vi "scale_matrix.vi"(1 "Scale Factors":cluster{dbl, dbl, dbl}) -> (0 "Scale Matrix":T1)   [LabVIEW 2019]
uses:
  <vilib>/Analysis/Matrix/Datatypes/RealMatrix.ctl
  <vilib>/Analysis/Matrix/Numeric/Conversions/Array To Matrix - RA2.vi
  <vilib>/Analysis/Matrix/NI_Matrix.lvlib
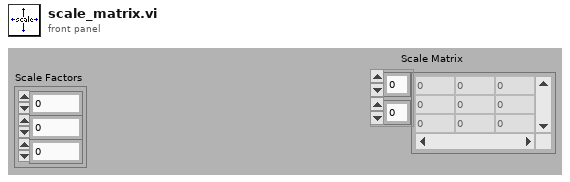
[diagram p1: front panel]
types:
  T1 = typedef "NI_Matrix.lvlib/RealMatrix.ctl" = dbl[][]
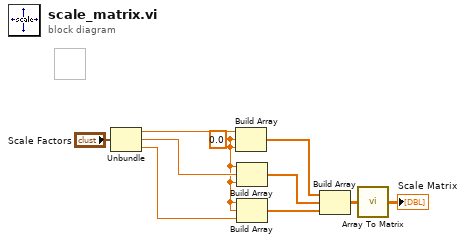
[diagram p0: block diagram]
diagram:
  w1 = 0.0 ("element")
  n1 = Unbundle("Scale Factors") -> (w4:dbl, w3:dbl, w2:dbl)
  n2 = Build Array(w4, w1, w1) -> (w9:dbl[])
  n3 = Build Array(w1, w3, w1) -> (w8:dbl[])
  n4 = Build Array(w1, w1, w2) -> (w7:dbl[])
  n5 = Build Array(w9, w8, w7) -> (w6:dbl[][])
  n6 = call-poly <vilib>:"Array To Matrix.vi"("Real 2D Array"=w6) -> ("Real Matrix"=→"Scale Matrix":T1)
